vi "TAT_Start.vi"(8 "error In":errorcluster) -> (0 "error out":errorcluster)   [LabVIEW 2017]
uses:
  <vilib>/addons/database/Connection.llb/Conn ObjectReference.ctl
  Controls/Ass. Loop Control.ctl
  <vilib>/Utility/error.llb/DialogType.ctl
  Controls/AUTO_STATE_QUEUE.ctl
  Global/PLC_to_Auto.vi
  <vilib>/addons/database/Connection.llb/DB Tools Open Connec (Path).vi
  <vilib>/addons/database/NI_Database_API.lvlib
panel:
  in  "Stop":bool
  out "DATE/TIME":string
  out "PLC 1 STATUS:-":bool
  out "Enum":T1
  out "BOX LH PART COUNT":string caption="BOX WEIGHT"
  out "BOX RH PART COUNT":string caption="BOX WEIGHT"
  out "FULL BOX WEIGHT":string caption="BOX WEIGHT"
  out "EMPTY BOX WEIGHT":string caption="BOX WEIGHT"
  out "USER :-":string
  out "RH SCAN CODE":string caption="SCAN CODE 1:-"
  out "Selected recipe":T2
  out "error in (no error) 3":errorcluster
  in  "error in (no error) 2":errorcluster
  out "FALSE healty":bool
  out "TRUE Duplication on Station 2":bool
  out "error out 2":errorcluster
  in  "Refnum in":T3
  out "Refnum out":T3
  in  "Scan Code":string
  in  "error in (no error)":errorcluster
  out "TRUE no barcode Done on station 1":bool
  out "Array 2":bool[](array[boolean])
  out "CYCLE STATUS STATION 2":string caption="CYCLE STATUS :-"
  in  "Tab Control":T4(tab)
  out "PLC HEALTHY:-":bool
  out "THREAD LOCKER CYC RUNNING:-":bool
  out "THREAD CYC AT HOME":bool
  out "PUSH AT HOME":bool
  out "DOOR 4":bool
  out "DOOR 3":bool
  out "DOOR 2":bool
  out "SAFETY SENSOR":bool
  out "PRESSURE SW":bool
  out "EMG":bool
  out "DOOR 1":bool
  out "alarms":string[](array[string])
  out "SHIFT :-":string
  out "CYCLE TIME :-":string
  out "NG COUNT :-":string
  out "OK COUNT :-":string
  out "PROJECT :-":string
  out "CYCLE STATUS STATION 1":string caption="CYCLE STATUS :-"
  out "LH SCAN CODE":string caption="SCAN CODE 1:-"
  # "AUTO CYCLE"
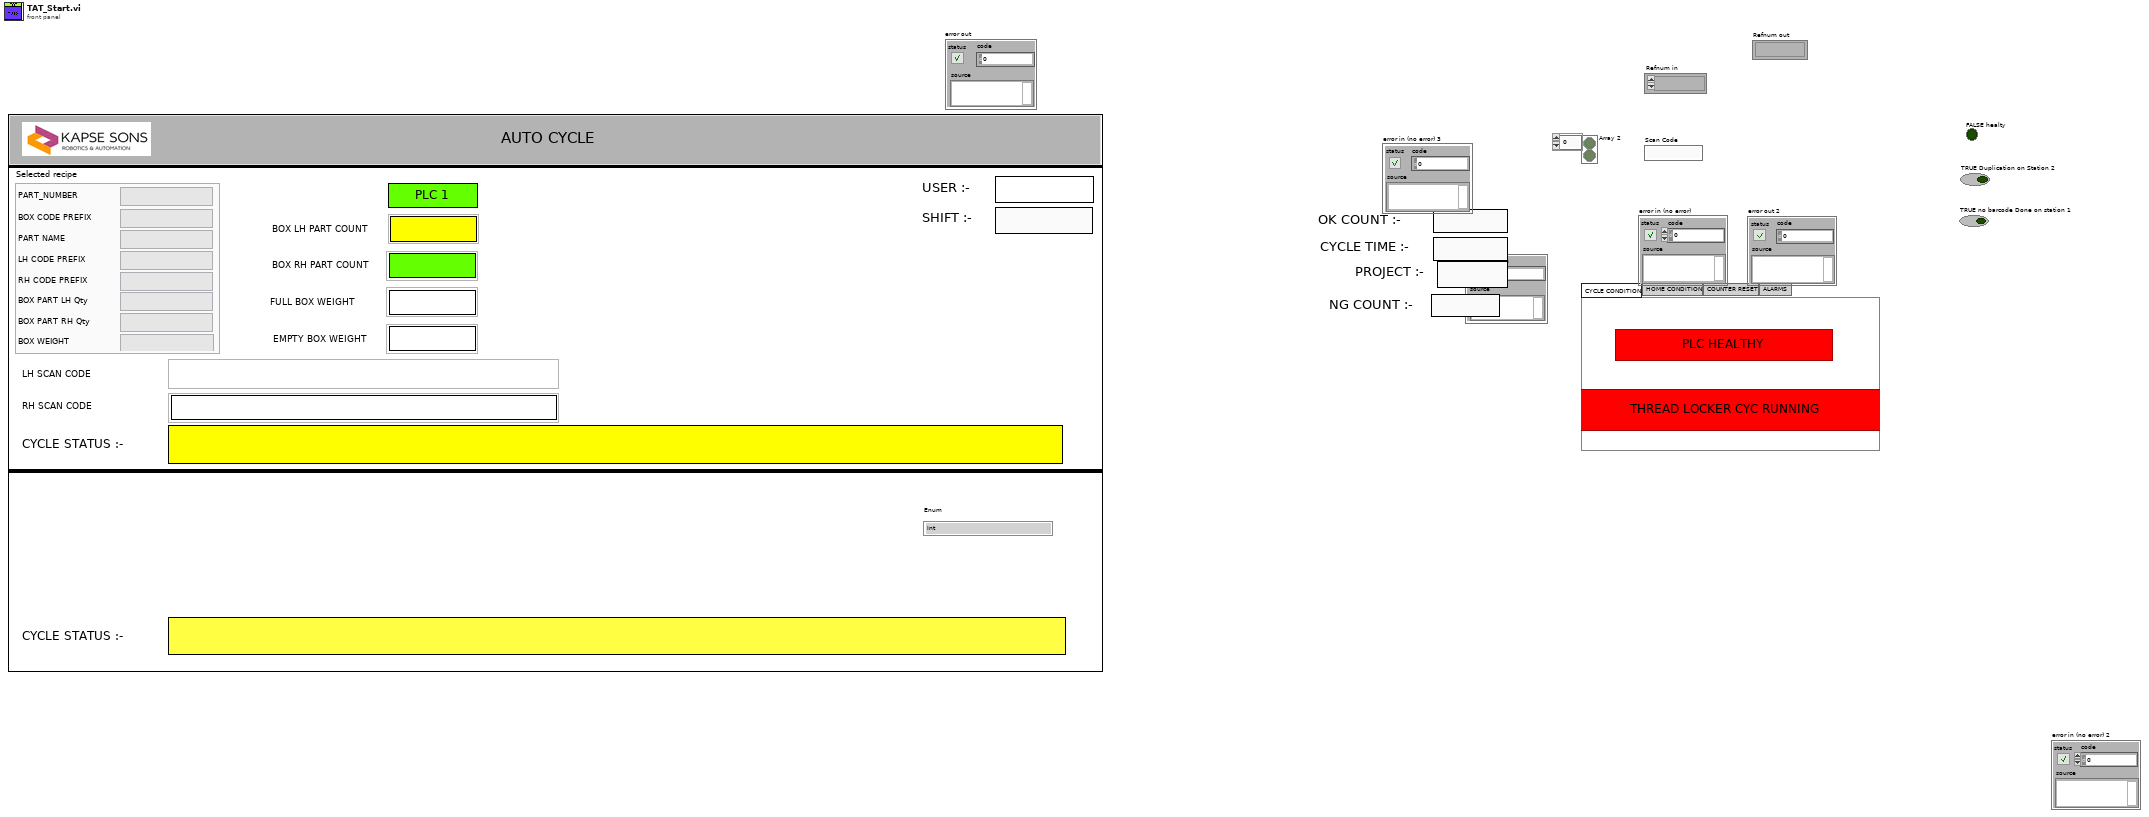
[diagram p1: front panel]
types:
  T1 = typedef "Ass. Loop Control.ctl" = enum16{"Int", "Int2", "Cluster_update", "Wait", "BOX_at_Filling_Station", "Scan_LH_Code", "Scan_RH_Code", "STATION1_Start Cycle", "STATION_1_SCAN", "STATION1_barcode CHECK", "STATION1_SaveDATA_sql", "STATION1_Cycle End", "STATION1_Cycle_Cancle", "STATION2_SCAN", "STATION2_SaveDATA_sql", "Stop", "Error Handler"}
  T2 = cluster{"PART_NUMBER":string, "BOX CODE PREFIX":string, "PART NAME":string, "LH CODE PREFIX":string, "RH CODE PREFIX":string, "BOX PART LH Qty":string, "BOX PART RH Qty":string, "BOX WEIGHT":string}
  T3 = typedef "NI_Database_API.lvlib/Conn ObjectReference.ctl" = refnum<k1>
  T4 = enum32{"CYCLE CONDITION", "HOME CONDITION", "COUNTER RESET", "ALARMS"}
  T5 = cluster{"SQL reference":T3, "RH Scanner Enable":bool, "LH Scanner Enable":bool, "Generated BOX QR code":string, "Selected recipe":cluster{"PART_NUMBER":string, "BOX CODE PREFIX":string, "PART NAME":string, "LH CODE PREFIX":string, "RH CODE PREFIX":string, "BOX PART LH Qty":string, "BOX PART RH Qty":string, "BOX WEIGHT":string}, "LH Scanner":refnum<k5>, "RH Scanner":refnum<k5>}
  T6 = typedef "AUTO_STATE_QUEUE.ctl" = enum16{"CREATE Q", "EN Q", "DE Q", "CLOSE Q"}
  T7 = typedef "DialogType.ctl" = u16
  T8 = enum32{"invalid app kind", "Development System", "Run Time System", "Student Edition", "Embedded LabVIEW", "Evaluation", "Custom"}
  T9 = cluster{"IP Address":string, "LH Scanner IP Address":string, "RH Scanner IP Address":string}
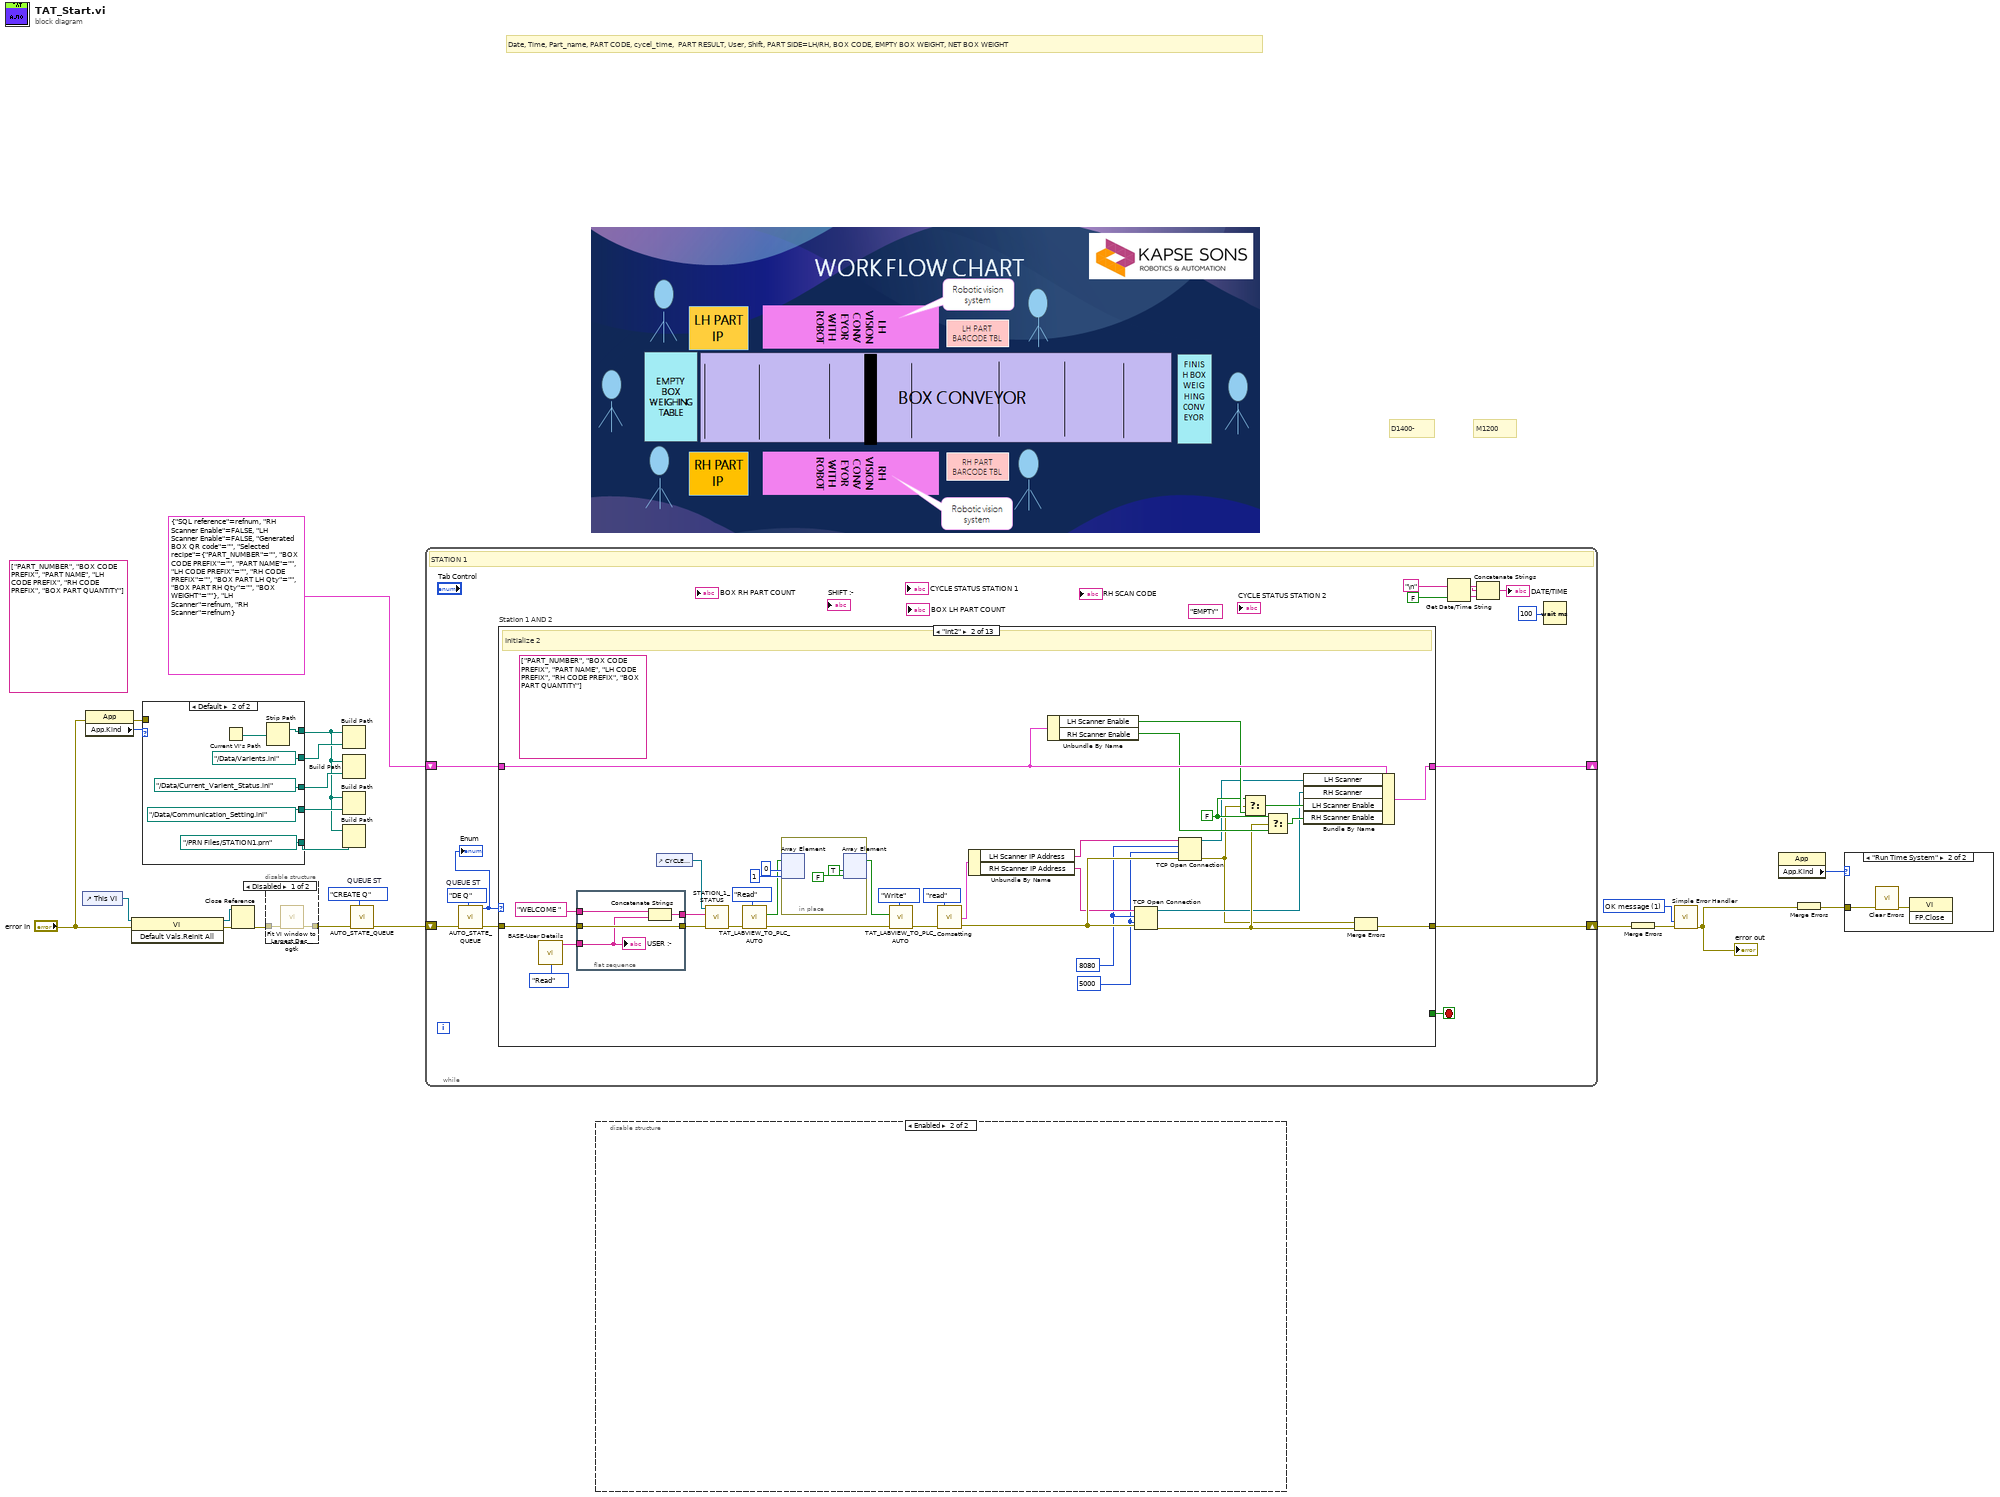
[diagram p0: block diagram]
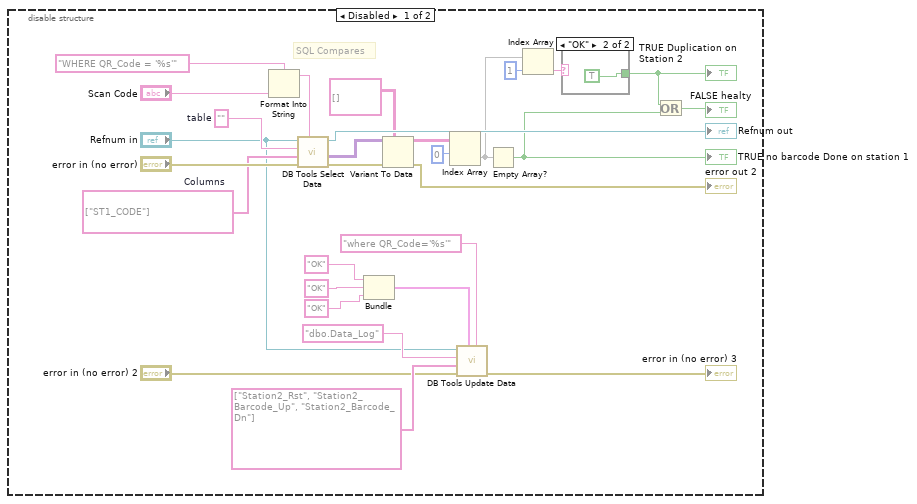
[diagram p2: hidden frame]
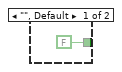
[diagram p3: hidden frame]
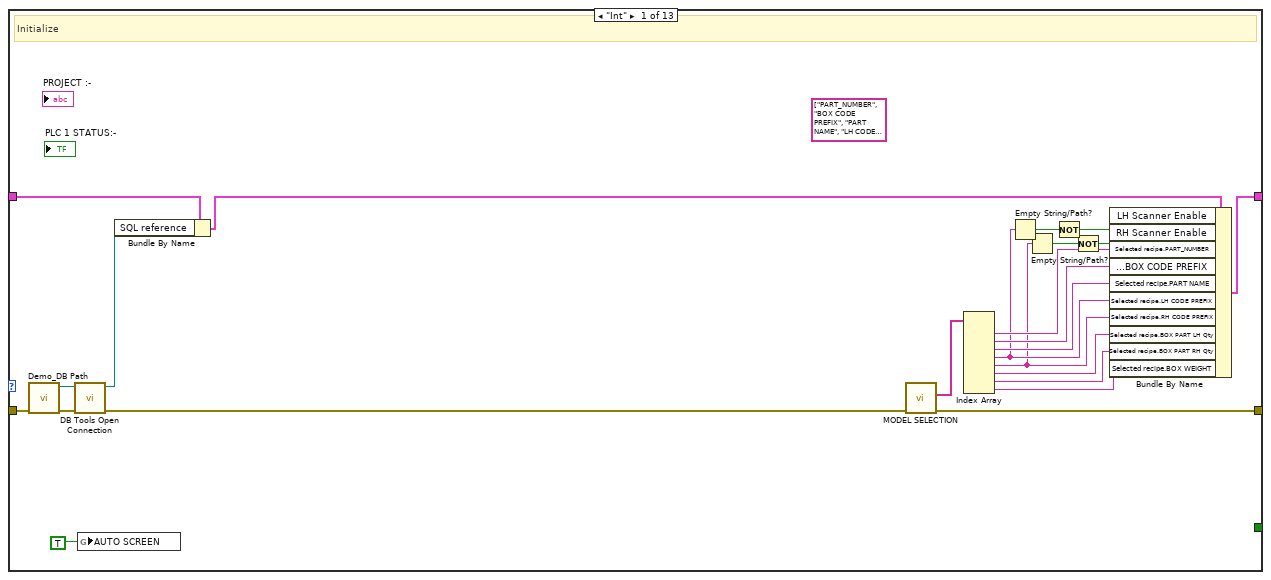
[diagram p6: hidden frame]
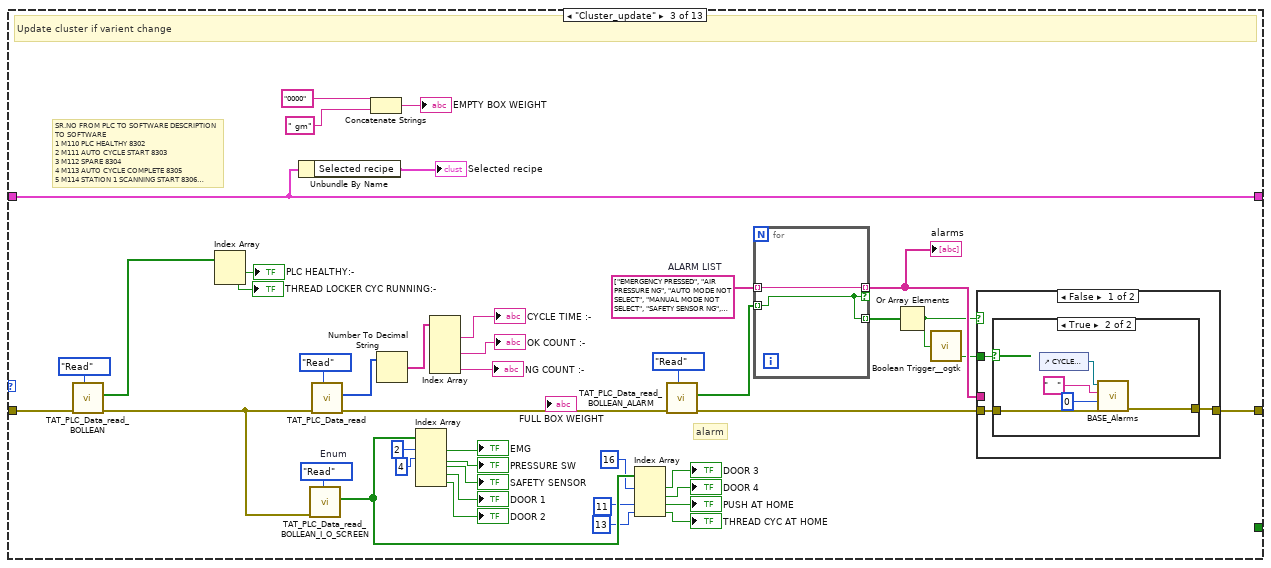
[diagram p7: hidden frame]
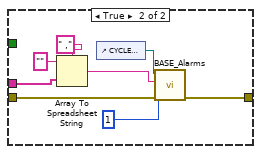
[diagram p9: hidden frame]
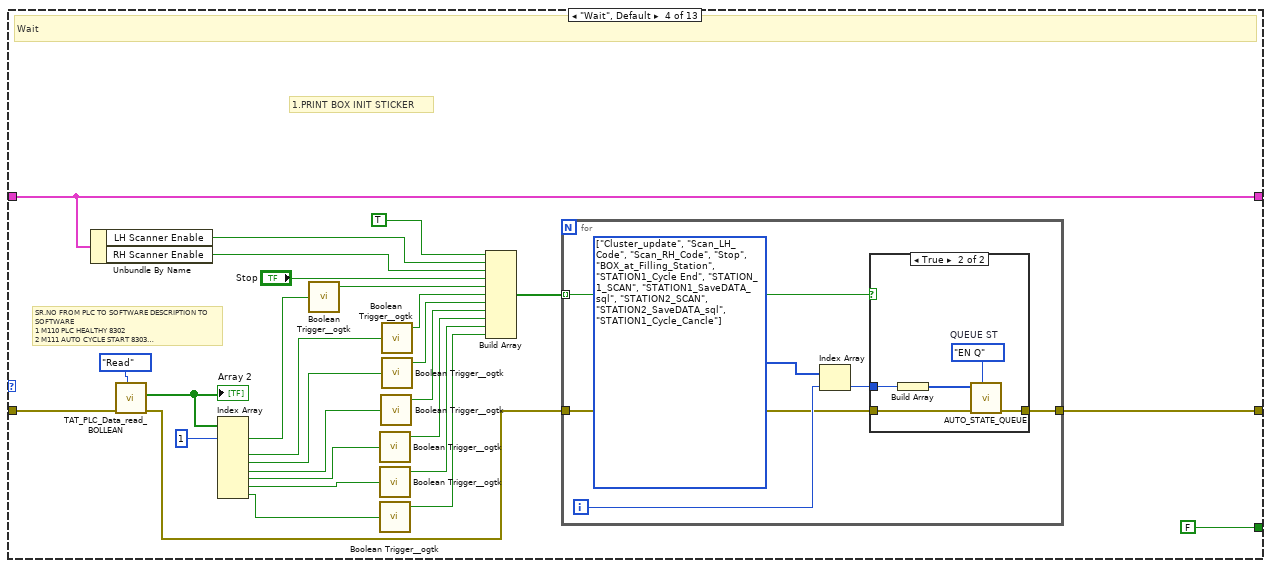
[diagram p10: hidden frame]
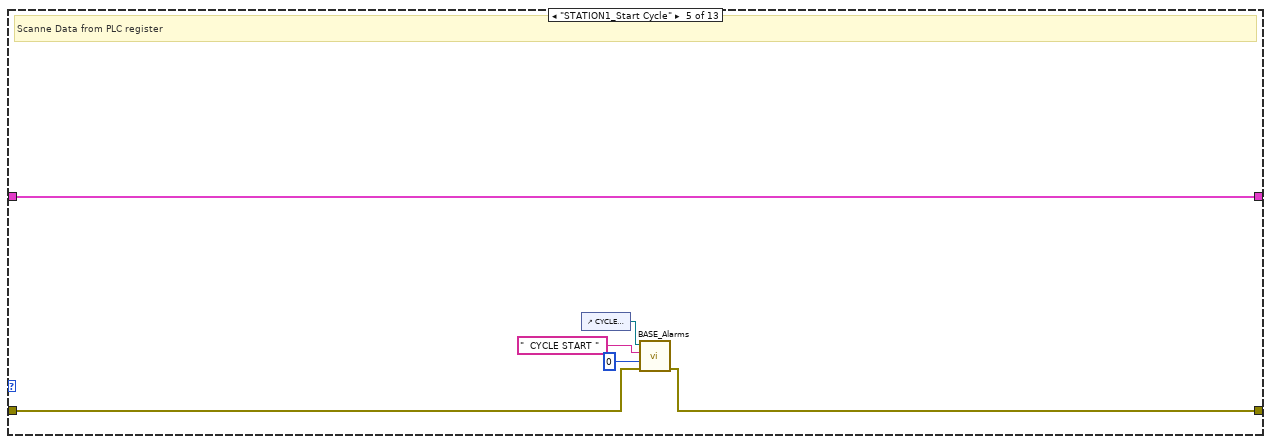
[diagram p12: hidden frame]
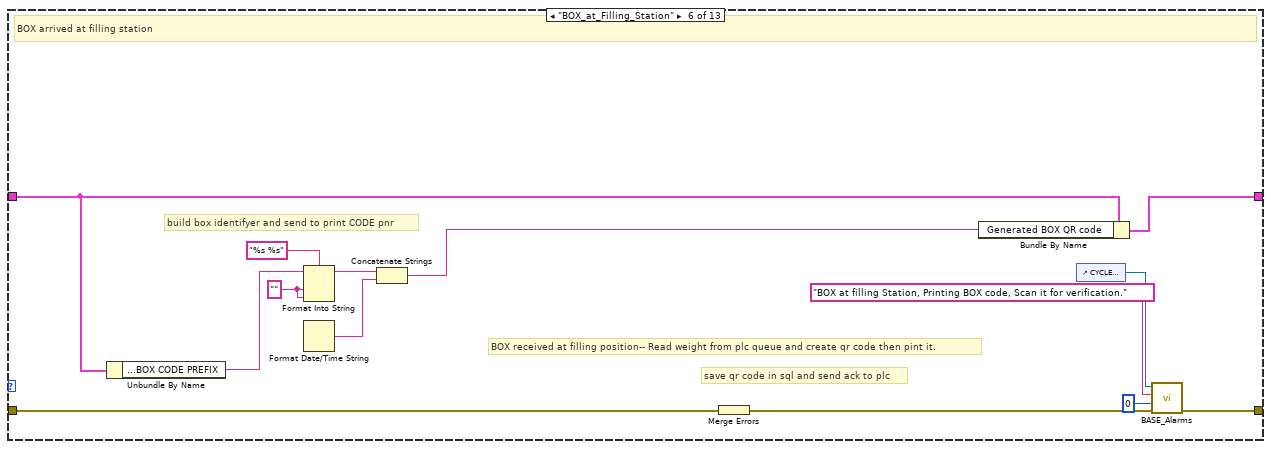
[diagram p13: hidden frame]
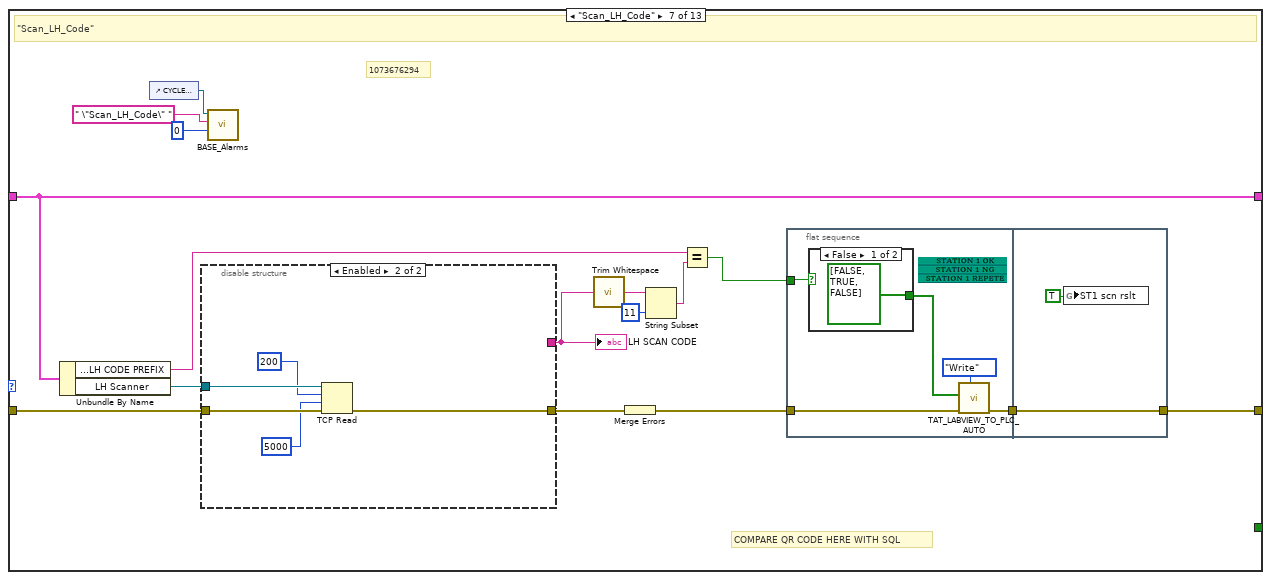
[diagram p14: hidden frame]
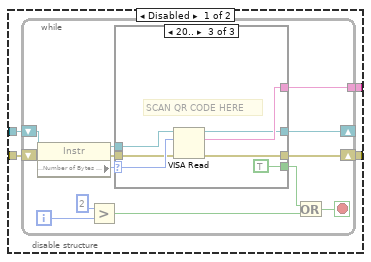
[diagram p15: hidden frame]
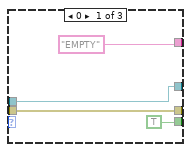
[diagram p16: hidden frame]
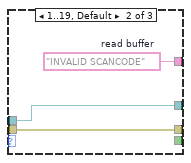
[diagram p17: hidden frame]
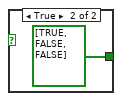
[diagram p18: hidden frame]
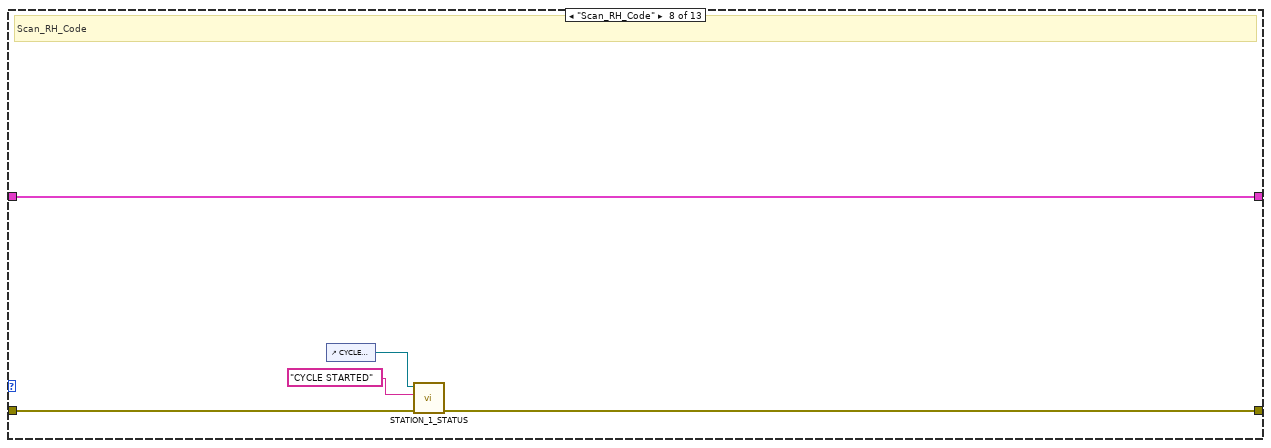
[diagram p19: hidden frame]
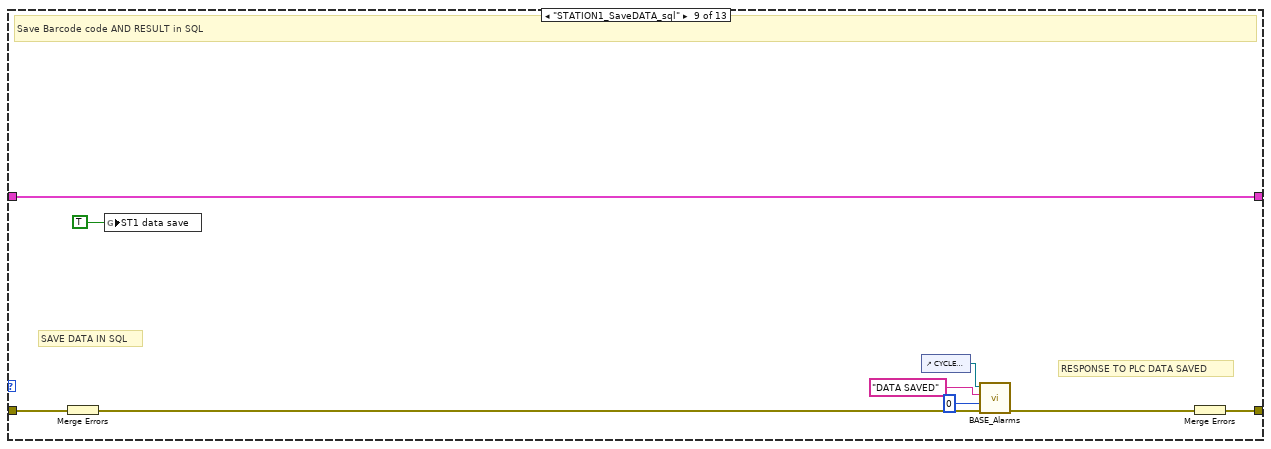
[diagram p20: hidden frame]
diagram:
  (unwired) string[] ["PART_NUMBER", "BOX CODE PREFIX", "PART NAME", "LH CODE PREFIX", "RH CODE PREFIX", "BOX PART QUANTITY"] ("Column Header Strings[]")
  w5 = AUTO_STATE_QUEUE."CREATE Q"  # QUEUE ST
  w17 = T7 1 items=["no dialog", "OK message", "continue or stop message", "OK message + warnings", "continue/stop + warnings"] ("type of dialog (OK msg:1)")
  # "M1200"
  # "D1400-"
  # "Date, Time, Part_name, PART CODE, cycel_time,  PART RESULT, User, Shift, PART SIDE=LH/RH, BOX CODE, EMPTY BOX WEIGHT, NET BOX WEIGHT"
  n1 = control-ref of="This VI"() -> (w22:refnum<vi>)
  n2 = property class="App"(error in="error In") -> (error out=w11:errorcluster, "App.Kind"=w15:T8)  [unwired: 1 in, 1 out]
  n3 = invoke class="VI" method="Default Vals.Reinit All"(reference=w22, error in="error In") -> (reference out=w20:refnum<vi>, error out=w21:errorcluster)  [unwired: 1 in, 1 out]
  n4 = case shown="Default" w15 {
    tunnel: [path "Data/Varients.ini" ("path") path "../Data/Varients.ini" ("path")] -> w14
    tunnel: [w26 w34] -> w6
    tunnel: [path "Data/Current_Varient_Status.ini" ("path") path "../Data/Current_Varient_Status.ini" ("path")] -> w13
    tunnel: [path "Data/Communication_Setting.ini" ("path") path "../Data/Communication_Setting.ini" ("path")] -> w12
    tunnel: w11 -> [_ _]
    tunnel: [path "PRN Files/STATION1.prn" ("path") path "../PRN Files/STATION1.prn" ("path")] -> w9
    frame "Run Time System" {
      n5 = Current VI's Path() -> (path=w29:path)
      n6 = Strip Path(path=w29) -> (stripped path=w28:path)  [unwired: 1 out]
      n7 = Strip Path(path=w28) -> (stripped path=w27:path)  [unwired: 1 out]
      n8 = Strip Path(path=w27) -> (stripped path=w26:path)  [unwired: 1 out]
    }
    frame Default {
      n9 = Current VI's Path() -> (path=w35:path)
      n10 = Strip Path(path=w35) -> (stripped path=w34:path)  [unwired: 1 out]
    }
  }
  n11 = Close Reference(reference=w20, error in (no error)=w21) -> (error out=w19:errorcluster)
  n12 = disable-structure shown="Disabled" {
    disable-tunnel: w19 -> [w38 w39]
    disable-tunnel: [w37 w39] -> w1
    frame Disabled {
      n13 = call <userlib>:"Fit VI window to Largest Dec__ogtk.vi"("error in (no error)"=w38) -> ("error out"=w37:errorcluster)  [unwired: 5 in, 1 out]
    }
    frame Enabled {
    }
  }
  n14 = Build Path(base path=w6, name or relative path=w14) -> ()  [unwired: 1 out]
  n15 = Build Path(base path=w6, name or relative path=w13) -> ()  [unwired: 1 out]
  n16 = Build Path(base path=w6, name or relative path=w12) -> ()  [unwired: 1 out]
  n17 = Build Path(base path=w6, name or relative path=w9) -> ()  [unwired: 1 out]
  n18 = call "AUTO_STATE_QUEUE.vi"("QUEUE ST"=w5, "error in"=w1) -> ("error OUT"=w4:errorcluster)  [unwired: 8 in, 1 out]
  n19 = while {
    shift-right: [w43] -> w3
    shift-left: w4 -> [w46]
    shift-right: [w42] -> _
    shift-left: T5 {"SQL reference"=refnum, "RH Scanner Enable"=FALSE, "LH Scanner Enable"=FALSE, "Generated BOX QR code"="", "Selected recipe"={"PART_NUMBER"="", "BOX CODE PREFIX"="", "PART NAME"="", "LH CODE PREFIX"="", "RH CODE PREFIX"="", "BOX PART LH Qty"="", "BOX PART RH Qty"="", "BOX WEIGHT"=""}, "LH Scanner"=refnum, "RH Scanner"=refnum} -> [w41]
    stop <- w47 stop-if-true
    (unwired) "EMPTY"
    w44 = AUTO_STATE_QUEUE."DE Q"  # QUEUE ST
    # "STATION 1"
    n20 = call "AUTO_STATE_QUEUE.vi"("QUEUE ST"=w44, "error in"=w46) -> ("error OUT"=w45:errorcluster, "Enum"=w40:T1)  [unwired: 8 in]
    "Enum" <- w40
    n21 = case "Station 1 AND 2" shown="\"Int2\"" w40 {
      tunnel: [_ _ _ FALSE _ _ _ _ _ _ _ _ TRUE] -> w47
      tunnel: [w69 w95 w145 w186 w221 w235 w251 w302 w311 w319 w327 w331 w344] -> w43
      tunnel: w45 -> [w62 w92 w159 w204 w219 w234 w253 w303 w313 w316 w325 w333 w346]
      tunnel: [w72 w91 w122 w182 w220 w226 w239 w300 w312 w314 w323 w330 w343] -> w42
      tunnel: w41 -> [w75 w90 w122 w182 w220 w227 w239 w300 w312 w315 w324 w330 w343]
      frame "Int" {
        (unwired) string[] ["PART_NUMBER", "BOX CODE PREFIX", "PART NAME", "LH CODE PREFIX", "RH CODE PREFIX", "BOX PART QUANTITY"] ("Column Header Strings[]")
        # "Initialize"
        n22 = call "Demo_DB Path.vi"("error in"=w62) -> ("error out"=w76:errorcluster, "DB Path"=w71:path)  [unwired: 9 in]
        n23 = call-poly <vilib>:"DB Tools Open Connection.vi"("error in (no error)"=w76, "connection information"=w71) -> ("error out"=w61:errorcluster, "connection reference"=w74:T3)  [unwired: 6 in]
        n24 = global write "PLC_to_Auto.vi" "AUTO SCREEN"(TRUE) -> ()
        n25 = Bundle By Name(cluster=w75, "SQL reference"=w74) -> (w73:T5)
        n26 = call "MODEL SELECTION.vi"("error in (no error)"=w61) -> ("error out 2"=w69:errorcluster, "qr code"=w68:string[])  [unwired: 8 in, 1 out]
        n27 = Index Array(array=w68) -> (element #1=w67:string, element #2=w66:string, element #3=w65:string, element #4=w60:string, element #5=w59:string, element #6=w64:string, element #7=w63:string, element #8=w54:string)  [unwired: 8 in]
        n28 = Empty String/Path?(string/path=w60) -> (empty?=w58:bool)
        n29 = Empty String/Path?(string/path=w59) -> (empty?=w57:bool)
        n30 = Not(x=w58) -> (.not. x?=w56:bool)
        n31 = Not(x=w57) -> (.not. x?=w55:bool)
        n32 = Bundle By Name(cluster=w73, "LH Scanner Enable"=w56, "RH Scanner Enable"=w55, "Selected recipe.PART_NUMBER"=w67, "Selected recipe.BOX CODE PREFIX"=w66, "Selected recipe.PART NAME"=w65, "Selected recipe.LH CODE PREFIX"=w60, "Selected recipe.RH CODE PREFIX"=w59, "Selected recipe.BOX PART LH Qty"=w64, "Selected recipe.BOX PART RH Qty"=w63, "Selected recipe.BOX WEIGHT"=w54) -> (w72:T5)
      }
      frame "Int2" {
        w77 = u16 5000 ("remote port or service name")
        w78 = u16 8080 ("remote port or service name")
        w86 = FALSE
        (unwired) string[] ["PART_NUMBER", "BOX CODE PREFIX", "PART NAME", "LH CODE PREFIX", "RH CODE PREFIX", "BOX PART QUANTITY"] ("Column Header Strings[]")
        # "Initialize 2"
        n33 = call "BASE-User Details.vi"("Enum"=enum16{"Read", "Write"}."Read") -> ("User Name Out"=w111:string)  [unwired: 9 in, 1 out]
        n34 = flat-sequence {
          tunnel: [w117] -> w108
          tunnel: w92 -> [w117]
          tunnel: w111 -> [w115]
          tunnel: "WELCOME " ("Cycle Status") -> [w116]
          tunnel: [w114] -> w106
          frame #0 {
            n35 = Concatenate Strings(w116, w115) -> (w114:string)
            "USER :-" <- w115
          }
        }
        n36 = control-ref of="CYCLE STATUS STATION 1"() -> (w109:refnum<vi>)
        n37 = call "STATION_1_STATUS.vi"("error in (no error)"=w108, "STATUS"=w106, "Ctl Refnum"=w109) -> ("error out"=w98:errorcluster)  [unwired: 8 in]
        n38 = call "TAT_LABVIEW_TO_PLC_AUTO.vi"("Enum"=enum16{"Read", "Write"}."Read", "error in (no error)"=w98) -> ("error out"=w97:errorcluster, "Array 2"=w99:bool[])  [unwired: 8 in]
        n39 = in-place {
          n40 = in-place-array #1(w99, 0, 1) -> ()  [unwired: 2 out]
          n41 = in-place-array #1(TRUE, FALSE) -> (w94:bool[])  [unwired: 2 out]
        }
        n42 = call "TAT_LABVIEW_TO_PLC_AUTO.vi"("Enum"=enum16{"Read", "Write"}."Write", "error in (no error)"=w97, "Array"=w94) -> ("error out"=w96:errorcluster)  [unwired: 7 in, 1 out]
        n43 = call "Comsetting.vi"("error in"=w96, "Enum"=enum16{"read", "write"}."read") -> ("error our"=w93:errorcluster, "Cluster Out"=w105:T9)  [unwired: 1 in, 1 out]
        n44 = Unbundle By Name(w105) -> ("LH Scanner IP Address"=w80:string, "RH Scanner IP Address"=w83:string)
        n45 = Unbundle By Name(w90) -> ("LH Scanner Enable"=w88:bool, "RH Scanner Enable"=w87:bool)
        n46 = TCP Open Connection(address=w83, remote port or service name=w78, timeout ms (60000)=w77, error in (no error)=w93) -> (connection ID=w82:refnum<k5>, error out=w84:errorcluster)  [unwired: 1 in]
        n47 = TCP Open Connection(address=w80, remote port or service name=w78, timeout ms (60000)=w77, error in (no error)=w93) -> (connection ID=w79:refnum<k5>, error out=w81:errorcluster)  [unwired: 1 in]
        n48 = Select(t=w86, s=w81, f=w88) -> (s? t:f=w89:bool)
        n49 = Select(t=w86, s=w84, f=w87) -> (s? t:f=w85:bool)
        n50 = Bundle By Name(cluster=w90, "LH Scanner"=w79, "RH Scanner"=w82, "LH Scanner Enable"=w89, "RH Scanner Enable"=w85) -> (w91:T5)
        n51 = Merge Errors(w81, w84) -> (w95:errorcluster)
      }
      frame "Cluster_update" {
        w140 = enum16{"Read", "Write"}."Read"  # Enum
        w148 = string[] ["EMERGENCY PRESSED", "AIR PRESSURE NG", "AUTO MODE NOT SELECT", "MANUAL MODE NOT SELECT", "SAFETY SENSOR NG", "TOUCH BUTTON NG", "PUSHER HOME RS NG", "PUSHER END RS NG", "THREAD LOCKER CYL HOME RS NG", "THREAD LOCKER CYL END RS NG", "PART CLAMP RS NG", "DOOR 1 NG", "DOOR 2 NG", "HOLE BLOCK", "SOFTWARE NOT RUN", "DOOR 3 NG", "DOOR 4 NG", "PART REJECT", "REJECTION BIN FULL"]  # ALARM LIST
        # "alarm"
        # "SR.NO\tFROM PLC TO SOFTWARE\tDESCRIPTION\tTO SOFTWARE\n1\tM110\tPLC HEALTHY\t8302\n2\tM111\tAUTO CYCLE START\t8303\n3\tM112\tSPARE\t8304\n4\tM113\tAUTO CYCLE COMPLETE\t8305\n5\tM114\tSTATION 1 SCANNING START\t8306\n6\tM115\tSTATION 1 DATA SAVE\t8307\n7\tM116\tSTATION 2 SCANNING START\t8308\n8\tM117\tSTATION 2 DATA SAVE\t8309"
        # "Update cluster if varient change"
        n52 = call "TAT_PLC_Data_read_BOLLEAN.vi"("Enum"=enum16{"Read", "Write"}."Read", "error in (no error)"=w159) -> ("error out"=w139:errorcluster, "Array 2"=w152:bool[])  [unwired: 8 in]
        n53 = Index Array(array=w152) -> (element #1=→"PLC HEALTHY:-":bool, element #2=→"THREAD LOCKER CYC RUNNING:-":bool)  [unwired: 2 in]
        n54 = Unbundle By Name(w122) -> ("Selected recipe"=→"Selected recipe":T2)
        n55 = call "TAT_PLC_Data_read_BOLLEAN_I_O_SCREEN.vi"("Enum"=w140, "error in (no error)"=w139) -> ("Array 2"=w131:bool[])  [unwired: 8 in, 1 out]
        n56 = call "TAT_PLC_Data_read.vi"("Enum"=enum16{"Read", "Write"}."Read", "error in (no error)"=w139) -> ("error out"=w149:errorcluster, "Array 2"=w157:u16[])  [unwired: 8 in]
        n57 = Concatenate Strings("0000", " gm") -> (→"EMPTY BOX WEIGHT":string)
        n58 = Number To Decimal String(number=w157) -> (decimal integer string=w156:string[])  [unwired: 1 in]
        n59 = Index Array(array=w131, index #1=2, index #2=4) -> (element #1=→"EMG":bool, element #2=→"PRESSURE SW":bool, element #3=→"SAFETY SENSOR":bool, element #4=→"DOOR 1":bool, element #5=→"DOOR 2":bool)  [unwired: 3 in]
        n60 = Index Array(array=w156) -> (element #1=→"CYCLE TIME :-":string, element #3=→"OK COUNT :-":string, element #5=→"NG COUNT :-":string)  [unwired: 5 in, 2 out]
        n61 = Index Array(array=w131, index #1=16, index #3=11, index #4=13) -> (element #1=→"DOOR 3":bool, element #2=→"DOOR 4":bool, element #3=→"PUSH AT HOME":bool, element #4=→"THREAD CYC AT HOME":bool)  [unwired: 1 in]
        n62 = call "TAT_PLC_Data_read_BOLLEAN_ALARM.vi"("Enum"=enum16{"Read", "Write"}."Read", "error in (no error)"=w149) -> ("error out"=w146:errorcluster, "Array 2"=w147:bool[])  [unwired: 8 in]
        n63 = for {
          tunnel: w148 -> [w179] mode=indexing
          tunnel: w147 -> [w178] mode=indexing
          tunnel: [w179] -> w143 mode=indexing if=w178
          tunnel: [w178] -> w144 mode=indexing
        }
        "alarms" <- w143
        n64 = Or Array Elements(Boolean array=w144) -> (logical OR=w142:bool)
        n65 = call <userlib>:"Boolean Trigger__ogtk.vi"("Boolean Input"=w142) -> ("Falling Edge"=w141:bool)  [unwired: 1 in, 1 out]
        n66 = case shown="False" w142 {
          tunnel: w146 -> [w161 w176]
          tunnel: [w162 w175] -> w145
          tunnel: w143 -> [_ w172]
          tunnel: w141 -> [w163 _]
          frame False {
            n67 = case shown="True" w163 {
              tunnel: [w164 w167] -> w162
              tunnel: w161 -> [w164 w166]
              frame False {
              }
              frame True {
                n68 = control-ref of="CYCLE STATUS STATION 1"() -> (w169:refnum<vi>)
                n69 = call "BASE_Alarms.vi"("error in (no error)"=w166, "FAULT NUMBER"=0, "STATUS"="   ", "Ctl Refnum"=w169) -> ("error out"=w167:errorcluster)  [unwired: 7 in]
              }
            }
          }
          frame True {
            n70 = Array To Spreadsheet String(delimiter (Tab)=" ,", array=w172, 3:"") -> (spreadsheet string=w171:string)
            n71 = control-ref of="CYCLE STATUS STATION 1"() -> (w177:refnum<vi>)
            n72 = call "BASE_Alarms.vi"("error in (no error)"=w176, "FAULT NUMBER"=1, "STATUS"=w171, "Ctl Refnum"=w177) -> ("error out"=w175:errorcluster)  [unwired: 7 in]
          }
        }
      }
      frame "Wait", Default {
        # "1.PRINT BOX INIT STICKER"
        # "SR.NO\tFROM PLC TO SOFTWARE\tDESCRIPTION\tTO SOFTWARE\n1\tM110\tPLC HEALTHY\t8302\n2\tM111\tAUTO CYCLE START\t8303\n3\tM112\tSPARE\t8304\n4\tM113\tAUTO CYCLE COMPLETE\t8305\n5\tM114\tSTATION 1 SCANNING START\t8306\n6\tM115\tSTATION 1 DATA SAVE\t8307\n7\tM116\tSTATION 2 SCANNING START\t8308\n8\tM117\tSTATION 2 DATA SAVE\t8309\n9 M118 Cycle Cancle St1 8310"
        # "Wait"
        n73 = Unbundle By Name(w182) -> ("LH Scanner Enable"=w180:bool, "RH Scanner Enable"=w181:bool)
        n74 = call "TAT_PLC_Data_read_BOLLEAN.vi"("Enum"=enum16{"Read", "Write"}."Read", "error in (no error)"=w204) -> ("error out"=w187:errorcluster, "Array 2"=w203:bool[])  [unwired: 8 in]
        "Array 2" <- w203
        n75 = Index Array(array=w203, index #1=1 ("index")) -> (element #1=w201:bool, element #3=w197:bool, element #4=w194:bool, element #5=w200:bool, element #6=w193:bool, element #7=w192:bool, element #8=w185:bool)  [unwired: 7 in, 1 out]
        n76 = call <userlib>:"Boolean Trigger__ogtk.vi"("Boolean Input"=w201) -> ("Rising Edge"=w199:bool)  [unwired: 1 in, 1 out]
        n77 = call <userlib>:"Boolean Trigger__ogtk.vi"("Boolean Input"=w193) -> ("Rising Edge"=w191:bool)  [unwired: 1 in, 1 out]
        n78 = call <userlib>:"Boolean Trigger__ogtk.vi"("Boolean Input"=w192) -> ("Rising Edge"=w190:bool)  [unwired: 1 in, 1 out]
        n79 = call <userlib>:"Boolean Trigger__ogtk.vi"("Boolean Input"=w185) -> ("Rising Edge"=w184:bool)  [unwired: 1 in, 1 out]
        n80 = call <userlib>:"Boolean Trigger__ogtk.vi"("Boolean Input"=w200) -> ("Rising Edge"=w195:bool)  [unwired: 1 in, 1 out]
        n81 = call <userlib>:"Boolean Trigger__ogtk.vi"("Boolean Input"=w197) -> ("Rising Edge"=w198:bool)  [unwired: 1 in, 1 out]
        n82 = call <userlib>:"Boolean Trigger__ogtk.vi"("Boolean Input"=w194) -> ("Rising Edge"=w196:bool)  [unwired: 1 in, 1 out]
        n83 = Build Array(TRUE, w180, w181, "Stop", w199, w198, w196, w195, w191, w190, w184) -> (w189:bool[])
        n84 = for {
          tunnel: w189 -> [w210] mode=indexing
          tunnel: w187 -> [w208]
          tunnel: [w207] -> w186
          i -> [w211]
          w212 = T1[] [enum."Cluster_update", enum."Scan_LH_Code", enum."Scan_RH_Code", enum."Stop", enum."BOX_at_Filling_Station", enum."STATION1_Cycle End", enum."STATION_1_SCAN", enum."STATION1_SaveDATA_sql", enum."STATION2_SCAN", enum."STATION2_SaveDATA_sql", enum."STATION1_Cycle_Cancle"] items=["Int", "Int2", "Cluster_update", "Wait", "BOX_at_Filling_Station", "Scan_LH_Code", "Scan_RH_Code", "STATION1_Start Cycle", "STATION_1_SCAN", "STATION1_barcode CHECK", "STATION1_SaveDATA_sql", "STATION1_Cycle End", "STATION1_Cycle_Cancle", "STATION2_SCAN", "STATION2_SaveDATA_sql", "Stop", "Error Handler"] ("Array")
          n85 = Index Array(array=w212, index=w211) -> (element=w209:T1)
          n86 = case shown="True" w210 {
            tunnel: w209 -> [_ w217]
            tunnel: w208 -> [w213 w215]
            tunnel: [w213 w214] -> w207
            frame False {
            }
            frame True {
              w218 = AUTO_STATE_QUEUE."EN Q"  # QUEUE ST
              n87 = Build Array(w217) -> (w216:T1[])
              n88 = call "AUTO_STATE_QUEUE.vi"("QUEUE ST"=w218, "error in"=w215, "AUTO ST"=w216) -> ("error OUT"=w214:errorcluster)  [unwired: 7 in, 1 out]
            }
          }
        }
      }
      frame "STATION1_Start Cycle" {
        # "Scanne Data from PLC register"
        n89 = control-ref of="CYCLE STATUS STATION 1"() -> (w224:refnum<vi>)
        n90 = call "BASE_Alarms.vi"("error in (no error)"=w219, "FAULT NUMBER"=0, "STATUS"="  CYCLE START ", "Ctl Refnum"=w224) -> ("error out"=w221:errorcluster)  [unwired: 7 in]
      }
      frame "BOX_at_Filling_Station" {
        w231 = ""
        # "BOX received at filling position-- Read weight from plc queue and create qr code then pint it."
        # "save qr code in sql and send ack to plc"
        # "build box identifyer and send to print CODE pnr"
        # "BOX arrived at filling station"
        n91 = Unbundle By Name(w227) -> ("Selected recipe.BOX CODE PREFIX"=w233:string)
        n92 = Format Into String(format string="%s %s", initial string=w233, w231, w231) -> (resulting string=w230:string)  [unwired: 1 in, 1 out]
        n93 = Format Date/Time String() -> (date/time string=w229:string)  [unwired: 3 in]
        n94 = Concatenate Strings(w230, w229) -> (w225:string)
        n95 = Merge Errors(w234) -> (w228:errorcluster)
        n96 = Bundle By Name(cluster=w227, "Generated BOX QR code"=w225) -> (w226:T5)
        n97 = control-ref of="CYCLE STATUS STATION 1"() -> (w238:refnum<vi>)
        n98 = call "BASE_Alarms.vi"("error in (no error)"=w228, "FAULT NUMBER"=0, "STATUS"="BOX at filling Station, Printing BOX code, Scan it for verification.", "Ctl Refnum"=w238) -> ("error out"=w235:errorcluster)  [unwired: 7 in]
      }
      frame "Scan_LH_Code" {
        # "1073676294"
        # "COMPARE QR CODE HERE WITH SQL"
        # "\"Scan_LH_Code\""
        n99 = Unbundle By Name(w239) -> ("Selected recipe.LH CODE PREFIX"=w244:string, "LH Scanner"=w254:refnum<k5>)
        n100 = control-ref of="CYCLE STATUS STATION 1"() -> (w249:refnum<vi>)
        n101 = disable-structure shown="Enabled" {
          disable-tunnel: w254 -> [w258 w288]
          disable-tunnel: w253 -> [w257 w290]
          disable-tunnel: [w256 w289] -> w252
          disable-tunnel: [w255 _] -> w246
          frame Disabled {
            n102 = while {
              shift-right: [w266] -> _
              shift-left: w258 -> [w270]
              shift-right: [w271] -> w256
              shift-left: w257 -> [w268]
              tunnel: [w259] -> w255
              i -> [w265]
              stop <- w261 stop-if-true
              n103 = property class="Instr"(reference=w270, error in=w268) -> (reference out=w269:refnum<visa-resource-name>, error out=w267:errorcluster, "Serial Settings:Number of Bytes at Serial Port"=w263:u32)
              n104 = Greater?(x=2 ("milliseconds to wait"), y=w265) -> (0:w262:bool)
              n105 = case shown="20.." w263 {
                selector: w263 -> [_ _ w285]
                tunnel: [w273 w276 w284] -> w271
                tunnel: w269 -> [w274 w277 w283]
                tunnel: w267 -> [w273 w276 w282]
                tunnel: ["EMPTY" w278 w281] -> w259
                tunnel: [w274 w277 w280] -> w266
                tunnel: [TRUE _ TRUE] -> w260
                frame 0 {
                }
                frame 1..19, Default {
                  w278 = "INVALID SCANCODE"  # read buffer
                }
                frame 20.. {
                  # "SCAN QR CODE HERE"
                  n106 = VISA Read(VISA resource name=w283, byte count=w285, error in (no error)=w282) -> (VISA resource name out=w280:refnum<visa-resource-name>, read buffer=w281:string, error out=w284:errorcluster)  [unwired: 1 out]
                }
              }
              n107 = Or(x=w260, y=w262) -> (x .or. y?=w261:bool)
            }
          }
          frame Enabled {
            n108 = TCP Read(connection ID=w288, bytes to read=200, error in (no error)=w290, 9:5000 ("timeout ms (25000)")) -> (error out=w289:errorcluster)  [unwired: 1 in, 2 out]
          }
        }
        "LH SCAN CODE" <- w246
        n109 = call "BASE_Alarms.vi"("FAULT NUMBER"=0, "STATUS"=" \"Scan_LH_Code\" ", "Ctl Refnum"=w249) -> ()  [unwired: 8 in, 1 out]
        n110 = call <vilib>:"Trim Whitespace.vi"("string"=w246) -> ("trimmed string"=w243:string)  [unwired: 1 in]
        n111 = Merge Errors(w252) -> (w240:errorcluster)
        n112 = String Subset(string=w243, length (rest)=11 ("length (rest)")) -> (substring=w242:string)  [unwired: 1 in]
        n113 = Equal?(x=w244, y=w242) -> (x = y?=w241:bool)
        n114 = flat-sequence {
          tunnel: w240 -> [w295]
          tunnel: [w293] -> w250
          tunnel: w241 -> [w292]
          tunnel: [w299] -> w251
          tunnel: w250 -> [w299]
          frame #0 {
            n115 = case shown="False" w292 {
              tunnel: [bool[] [FALSE, TRUE, FALSE] bool[] [TRUE, FALSE, FALSE]] -> w291
              frame False {
              }
              frame True {
              }
            }
            n116 = call "TAT_LABVIEW_TO_PLC_AUTO.vi"("Enum"=enum16{"Read", "Write"}."Write", "error in (no error)"=w295, "Array"=w291) -> ("error out"=w293:errorcluster)  [unwired: 7 in, 1 out]
          }
          frame #1 {
            n117 = global write "PLC_to_Auto.vi" "ST1 scn rslt"(TRUE) -> ()
          }
        }
      }
      frame "Scan_RH_Code" {
        # "Scan_RH_Code"
        n118 = control-ref of="CYCLE STATUS STATION 1"() -> (w301:refnum<vi>)
        n119 = call "STATION_1_STATUS.vi"("error in (no error)"=w303, "STATUS"="CYCLE STARTED" ("Cycle Status"), "Ctl Refnum"=w301) -> ("error out"=w302:errorcluster)  [unwired: 8 in]
      }
      frame "STATION1_SaveDATA_sql" {
        # "RESPONSE TO PLC DATA SAVED"
        # "SAVE DATA IN SQL"
        # "Save Barcode code AND RESULT in SQL"
        n120 = Merge Errors(w313) -> (w306:errorcluster)
        n121 = global write "PLC_to_Auto.vi" "ST1 data save"(TRUE) -> ()
        n122 = control-ref of="CYCLE STATUS STATION 1"() -> (w309:refnum<vi>)
        n123 = call "BASE_Alarms.vi"("error in (no error)"=w306, "FAULT NUMBER"=0, "STATUS"="DATA SAVED", "Ctl Refnum"=w309) -> ("error out"=w305:errorcluster)  [unwired: 7 in]
        n124 = Merge Errors(w305) -> (w311:errorcluster)
      }
      frame "STATION1_Cycle End" {
        # "CYCLE END"
        # "STATION 1 CYCLE END"
        n125 = Unbundle By Name(w315) -> ("LH Scanner"=w317:refnum<k5>)
        n126 = Merge Errors(w316) -> (w318:errorcluster)
        n127 = Bundle By Name(cluster=w315, "LH Scanner"=w317) -> (w314:T5)
        n128 = control-ref of="CYCLE STATUS STATION 1"() -> (w321:refnum<vi>)
        n129 = call "STATION_1_STATUS.vi"("error in (no error)"=w318, "STATUS"="CYCLE END" ("Cycle Status"), "Ctl Refnum"=w321) -> ("error out"=w319:errorcluster)  [unwired: 8 in]
      }
      frame "STATION1_Cycle_Cancle" {
        # "CYCLE END"
        # "STATION 1 CYCLE CANCLE"
        n130 = Unbundle By Name(w324) -> ("LH Scanner Enable"=w322:bool)
        n131 = Bundle By Name(cluster=w324, "LH Scanner Enable"=w322) -> (w323:T5)
        n132 = Merge Errors(w325) -> (w326:errorcluster)
        n133 = control-ref of="CYCLE STATUS STATION 1"() -> (w329:refnum<vi>)
        n134 = call "STATION_1_STATUS.vi"("error in (no error)"=w326, "STATUS"="CYCLE CANCLE" ("Cycle Status"), "Ctl Refnum"=w329) -> ("error out"=w327:errorcluster)  [unwired: 8 in]
      }
      frame "Error Handler" {
        w334 = T7 2 items=["no dialog", "OK message", "continue or stop message", "OK message + warnings", "continue/stop + warnings"] ("type of dialog (OK msg:1)")
        # "error handling"
        n135 = call <vilib>:"Simple Error Handler.vi"("type of dialog (OK msg:1)"=w334, "error in (no error)"=w333) -> ("error out"=w332:errorcluster)  [unwired: 3 in, 4 out]
        n136 = call <vilib>:"Clear Errors.vi"("error in (no error)"=w332) -> ("error out"=w331:errorcluster)  [unwired: 5 in, 1 out]
      }
      frame "Stop" {
        n137 = Unbundle By Name(w343) -> ("RH Scanner"=w335:refnum<k5>, "LH Scanner"=w337:refnum<k5>, "SQL reference"=w340:T3)
        n138 = control-ref of="CYCLE STATUS STATION 1"() -> (w345:refnum<vi>)
        n139 = call "STATION_1_STATUS.vi"("error in (no error)"=w346, "STATUS"="STOP" ("Cycle Status"), "Ctl Refnum"=w345) -> ("error out"=w344:errorcluster)  [unwired: 8 in]
        n140 = call <vilib>:"Clear Errors.vi"("error in (no error)"=w344) -> ("error out"=w341:errorcluster)  [unwired: 5 in, 1 out]
        n141 = Not A Number/Path/Refnum?(number/path/refnum=w340) -> (NaN/Path/Refnum?=w339:bool)
        n142 = Not A Number/Path/Refnum?(number/path/refnum=w337) -> (NaN/Path/Refnum?=w338:bool)
        n143 = Not A Number/Path/Refnum?(number/path/refnum=w335) -> (NaN/Path/Refnum?=w336:bool)
        n144 = case shown="False" w339 {
          tunnel: w340 -> [w354 _]
          tunnel: w341 -> [w353 _]
          frame False {
            n145 = call <vilib>:"DB Tools Close Connection.vi"("error in (no error)"=w353, "connection reference"=w354) -> ()  [unwired: 5 in, 1 out]
          }
          frame True {
          }
        }
        n146 = case shown="False" w336 {
          tunnel: w341 -> [w349 _]
          tunnel: w335 -> [w350 _]
          frame False {
            n147 = TCP Close Connection(connection ID=w350, error in (no error)=w349) -> ()  [unwired: 1 in, 2 out]
          }
          frame True {
          }
        }
        n148 = case shown="False" w338 {
          tunnel: w341 -> [w352 _]
          tunnel: w337 -> [w351 _]
          frame False {
            n149 = TCP Close Connection(connection ID=w351, error in (no error)=w352) -> ()  [unwired: 1 in, 2 out]
          }
          frame True {
          }
        }
        n150 = global write "PLC_to_Auto.vi" "AUTO SCREEN"(FALSE) -> ()
      }
    }
    n151 = Get Date/Time String(want seconds? (F)=FALSE) -> (date string=w51:string, time string=w50:string)  [unwired: 2 in]
    n152 = Concatenate Strings(w51, "\n", w50) -> (→"DATE/TIME":string)
    n153 = Wait (ms)(milliseconds to wait=u32 100) -> ()  [unwired: 1 out]
  }
  n154 = disable-structure shown="Enabled" {
    frame Disabled {
      w379 = string[] ["ST1_CODE"]  # Columns
      w380 = ""  # table
      # "SQL Compares"
      n155 = Format Into String(format string="WHERE QR_Code = '%s'", "Scan Code") -> (resulting string=w365:string)  [unwired: 2 in, 1 out]
      n156 = call <vilib>:"DB Tools Select Data.vi"("condition"=w365, "error in (no error)"="error in (no error)", "columns"=w379, "table"=w380, "connection reference"="Refnum in") -> ("error out"=w374:errorcluster, "data"=w376:variant[][], "connection reference out"=→"Refnum out":T3)  [unwired: 1 in]
      n157 = Bundle("OK", "OK", "OK") -> (w362:cluster{string, string, string})  [unwired: 1 in]
      n158 = Variant To Data(error in=w374, type=string[][] [], Variant=w376) -> (data=w375:string[][], error out=→"error out 2":errorcluster)
      n159 = Index Array(array=w375, index (row)=0) -> (element=w372:string[])  [unwired: 1 in]
      n160 = call <vilib>:"DB Tools Update Data.vi"("condition"="where QR_Code='%s'" ("format string"), "data"=w362, "error in (no error)"="error in (no error) 2", "columns"=string[] ["Station2_Rst", "Station2_Barcode_Up", "Station2_Barcode_Dn"] ("columns 2"), "table"="dbo.Data_Log", "connection reference"="Refnum in") -> ("error out"=→"error in (no error) 3":errorcluster)  [unwired: 4 in, 1 out]
      n161 = Empty Array?(array=w372) -> (empty?=w369:bool)
      "TRUE no barcode Done on station 1" <- w369
      n162 = Index Array(array=w372, index=1 ("index (row)")) -> (element=w371:string)
      n163 = case shown="\"OK\"" w371 {
        tunnel: [FALSE TRUE] -> w368
        frame "", Default {
        }
        frame "OK" {
        }
      }
      "TRUE Duplication on Station 2" <- w368
      n164 = Or(x=w368, y=w369) -> (x .or. y?=→"FALSE healty":bool)
    }
    frame Enabled {
    }
  }
  n165 = Merge Errors(w3) -> (w18:errorcluster)
  n166 = call <vilib>:"Simple Error Handler.vi"("type of dialog (OK msg:1)"=w17, "error in (no error)"=w18) -> ("error out"=w7:errorcluster)  [unwired: 3 in, 4 out]
  "error out" <- w7
  n167 = property class="App"() -> ("App.Kind"=w16:T8)  [unwired: 2 in, 2 out]
  n168 = Merge Errors(w7) -> (w8:errorcluster)
  n169 = case shown="\"Run Time System\"" w16 {
    tunnel: w8 -> [_ w387]
    frame "invalid app kind", Default {
    }
    frame "Run Time System" {
      n170 = call <vilib>:"Clear Errors.vi"("error in (no error)"=w387) -> ("error out"=w386:errorcluster)  [unwired: 5 in, 1 out]
      n171 = invoke class="VI" method="FP.Close"(error in=w386) -> ()  [unwired: 2 in, 3 out]
    }
  }
